vi "Program Setup.vi"(8 "error in (no error)":errorcluster, 10 "shutdown":refnum<user-event>, 11 "Modules":T9) -> (0 "error out":errorcluster)   [LabVIEW 2025]
uses:
  Controls/Sequencer/sequence array.ctl
  Controls/Sequencer/step cluster.ctl
  Controls/Sequencer/action enum.ctl
  Controls/Sequencer/plus button.ctl
  Controls/Sequencer/delete button.ctl
  Controls/Sequencer/save icon.ctl
  Controls/transparent tab control.ctl
  Controls/refresh button 2.ctl
  <vilib>/Handler Framework/CmdQueue/Enqueue Single.vi
  <vilib>/Handler Framework/Handler Framework.lvlib
panel:
  in  "Tab Control":T1
  in  "Refresh":T2
  in  "Program":u16(ring) items=["145", "156", "157", "166", "178"]
  out "View Program Array":T3=[{"Action"=enum."Start", "Angle Min [°]"=0.0, "Angle Max [°]"=0.0, "Torque Min [oz-in]"=0.0, "Torque Max [oz-in]"=0.0}, {"Action"=enum."Return to Home", "Angle Min [°]"=0.0, "Angle Max [°]"=0.0, "Torque Min [oz-in]"=0.0, "Torque Max [oz-in]"=0.0}, {"Action"=enum."End", "Angle Min [°]"=0.0, "Angle Max [°]"=0.0, "Torque Min [oz-in]"=0.0, "Torque Max [oz-in]"=0.0}]
  in  "Array":T3=[{"Action"=enum."Start", "Angle Min [°]"=0.0, "Angle Max [°]"=0.0, "Torque Min [oz-in]"=0.0, "Torque Max [oz-in]"=0.0}, {"Action"=enum."Return to Home", "Angle Min [°]"=0.0, "Angle Max [°]"=0.0, "Torque Min [oz-in]"=0.0, "Torque Max [oz-in]"=0.0}, {"Action"=enum."End", "Angle Min [°]"=0.0, "Angle Max [°]"=0.0, "Torque Min [oz-in]"=0.0, "Torque Max [oz-in]"=0.0}]
  in  "Add Step":T6
  in  "Delete Step":T7
  in  "Save Program":T8
  # "Edit Programs"
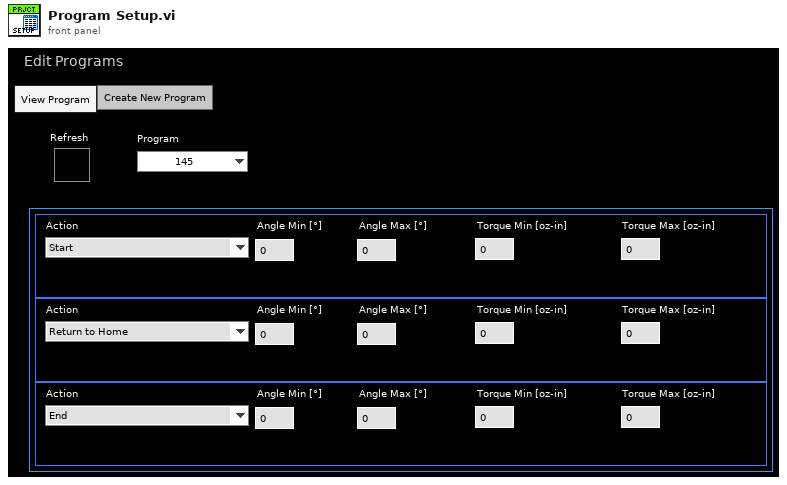
[diagram p1: front panel]
types:
  T1 = typedef "transparent tab control.ctl" = enum32{"View Program", "Create New Program"}
  T2 = typedef "refresh button 2.ctl" = bool
  T3 = typedef "sequence array.ctl" = T4[]
  T4 = typedef "step cluster.ctl" = cluster{"Action":T5, "Angle Min [°]":dbl, "Angle Max [°]":dbl, "Torque Min [oz-in]":dbl, "Torque Max [oz-in]":dbl}
  T5 = typedef "action enum.ctl" = enum16{"Start", "Angle", "Return to Home", "End"}
  T6 = typedef "plus button.ctl" = bool
  T7 = typedef "delete button.ctl" = bool
  T8 = typedef "save icon.ctl" = bool
  T9 = cluster{"Module IDs":i32[], "Module Names":string[]}
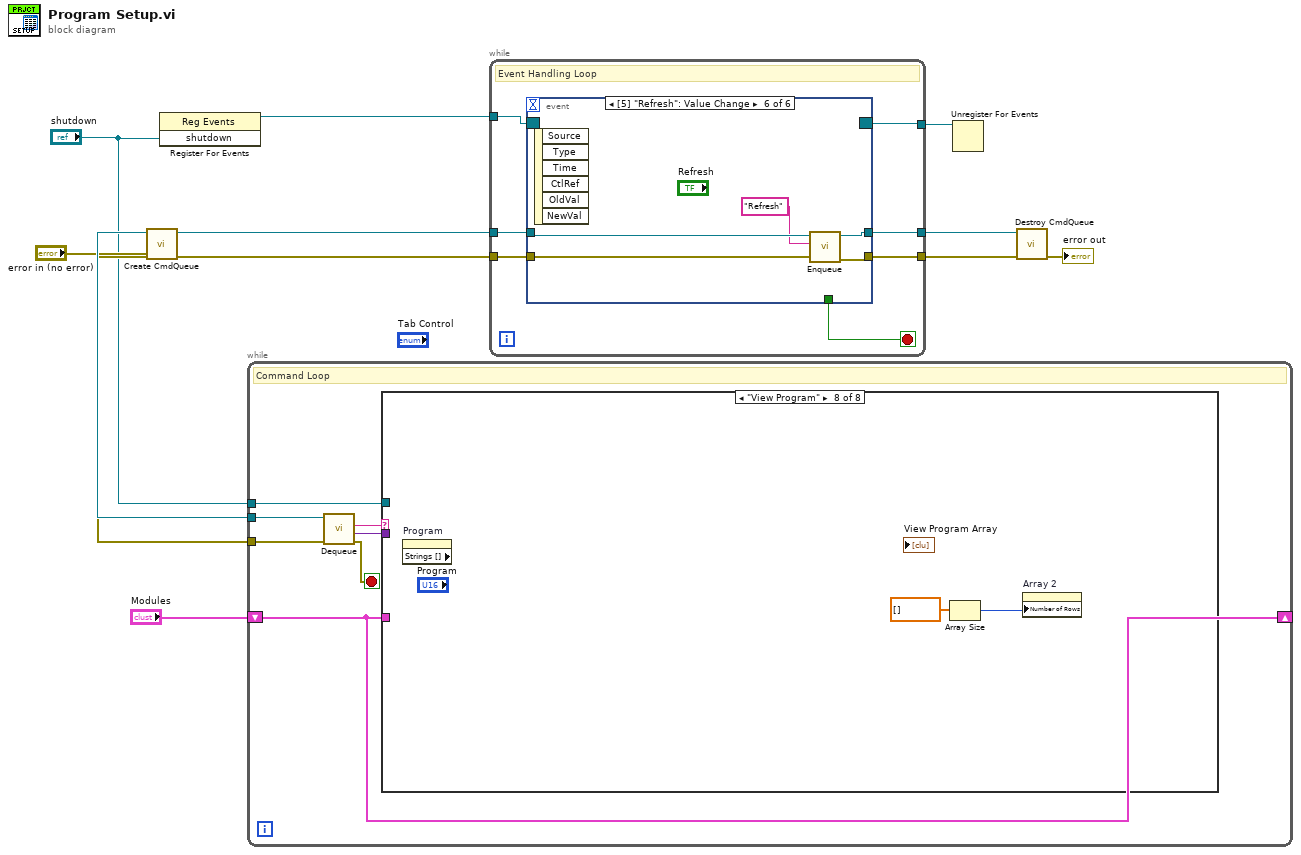
[diagram p0: block diagram]
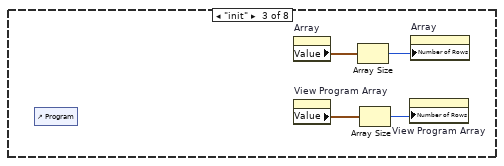
[diagram p4: hidden frame]
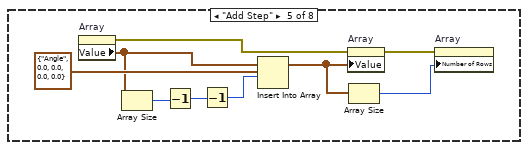
[diagram p6: hidden frame]
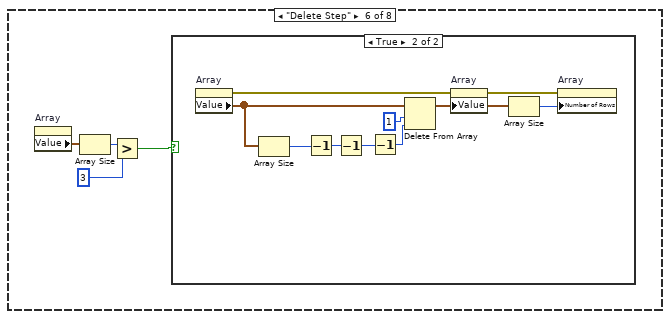
[diagram p7: hidden frame]
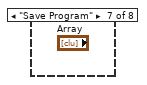
[diagram p9: hidden frame]
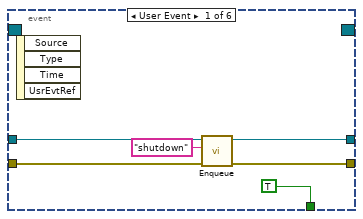
[diagram p10: hidden frame]
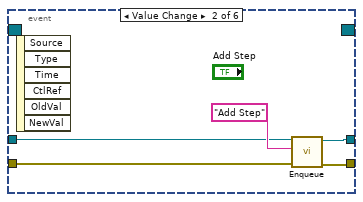
[diagram p11: hidden frame]
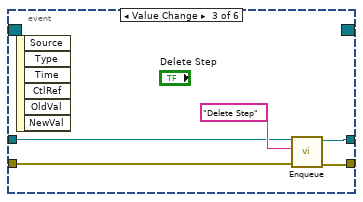
[diagram p12: hidden frame]
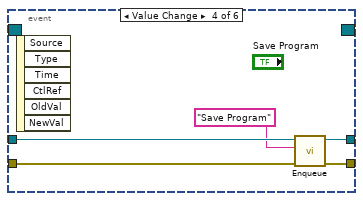
[diagram p13: hidden frame]
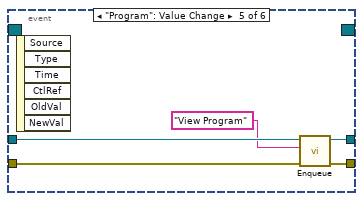
[diagram p14: hidden frame]
diagram:
  n1 = call <vilib>:"Create CmdQueue.vi"("error in (no error)"="error in (no error)") -> ("error out"=w7:errorcluster, "CmdQueue out"=w8:refnum<queue>)  [unwired: 9 in]
  n2 = register-events("shutdown") -> (reference out=w6:refnum<event-registration>)  [unwired: 2 in, 1 out]
  n3 = while {
    tunnel: w8 -> [w17]
    tunnel: w7 -> [w13]
    tunnel: "shutdown" -> [w12]
    shift-right: [w11] -> _
    shift-left: "Modules" -> [w11]
    stop <- w14 stop-if-true
    # "Command Loop"
    n4 = call <vilib>:"Dequeue.vi"("error in (no error)"=w13, "CmdQueue in"=w17) -> ("error out"=w14:errorcluster, "value"=w15:variant, "cmd"=w16:string)  [unwired: 5 in, 2 out]
    n5 = case shown="\"View Program\"" w16 {
      tunnel: w15 -> [_ _ _ _ _ _ _ _]
      tunnel: w12 -> [_ _ _ _ _ _ _ _]
      tunnel: w11 -> [_ _ _ _ _ _ _ _]
      frame "False", Default {
      }
      frame "Refresh" {
      }
      frame "init" {
        n6 = control-ref of="Program"() -> ()  [unwired: 1 out]
        n7 = property on="Array" class="Arr (strict)"() -> ("Value"=w18:T3)  [unwired: 2 in, 2 out]
        n8 = property on="View Program Array" class="Arr (strict)"() -> ("Value"=w20:T3)  [unwired: 2 in, 2 out]
        n9 = Array Size(array=w18) -> (size(s)=w19:i32)
        n10 = Array Size(array=w20) -> (size(s)=w21:i32)
        n11 = property on="View Program Array" class="Arr (strict)"("Number of Rows"=w21) -> ()  [unwired: 2 in, 2 out]
        n12 = property on="Array" class="Arr (strict)"("Number of Rows"=w19) -> ()  [unwired: 2 in, 2 out]
      }
      frame "shutdown" {
      }
      frame "Add Step" {
        n13 = property on="Array" class="Arr (strict)"() -> (error out=w30:errorcluster, "Value"=w23:T3)  [unwired: 2 in, 1 out]
        n14 = Array Size(array=w23) -> (size(s)=w22:i32)
        n15 = Decrement(x=w22) -> (x-1=w29:i32)
        n16 = Decrement(x=w29) -> (x-1=w28:i32)
        n17 = Insert Into Array(array=w23, index=w28, new element=T4 {"Action"=enum."Angle", "Angle Min [°]"=0.0, "Angle Max [°]"=0.0, "Torque Min [oz-in]"=0.0, "Torque Max [oz-in]"=0.0} ("new element/subarray")) -> (w26:T3)
        n18 = property on="Array" class="Arr (strict)"(error in=w30, "Value"=w26) -> (error out=w27:errorcluster)  [unwired: 1 in, 1 out]
        n19 = Array Size(array=w26) -> (size(s)=w25:i32)
        n20 = property on="Array" class="Arr (strict)"(error in=w27, "Number of Rows"=w25) -> ()  [unwired: 1 in, 2 out]
      }
      frame "Delete Step" {
        n21 = property on="Array" class="Arr (strict)"() -> ("Value"=w34:T3)  [unwired: 2 in, 2 out]
        n22 = Array Size(array=w34) -> (size(s)=w33:i32)
        n23 = Greater?(x=w33, y=3) -> (0:w31:bool)
        n24 = case shown="True" w31 {
          frame False {
          }
          frame True {
            n25 = property on="Array" class="Arr (strict)"() -> (error out=w43:errorcluster, "Value"=w37:T3)  [unwired: 2 in, 1 out]
            n26 = Array Size(array=w37) -> (size(s)=w35:i32)
            n27 = Decrement(x=w35) -> (x-1=w36:i32)
            n28 = Decrement(x=w36) -> (x-1=w42:i32)
            n29 = Decrement(x=w42) -> (x-1=w41:i32)
            n30 = Delete From Array(array=w37, length=1, index=w41) -> (array with subset deleted=w39:T3)  [unwired: 1 out]
            n31 = property on="Array" class="Arr (strict)"(error in=w43, "Value"=w39) -> (error out=w40:errorcluster)  [unwired: 1 in, 1 out]
            n32 = Array Size(array=w39) -> (size(s)=w38:i32)
            n33 = property on="Array" class="Arr (strict)"(error in=w40, "Number of Rows"=w38) -> ()  [unwired: 1 in, 2 out]
          }
        }
      }
      frame "Save Program" {
      }
      frame "View Program" {
        n34 = property on="Program" class="Ring (strict)" props=["Strings []"]() -> ()  [unwired: 2 in, 3 out]
        n35 = Array Size(array=dbl[] []) -> (size(s)=w46:i32)
        n36 = property on="Array 2" class="Arr (strict)"("Number of Rows"=w46) -> ()  [unwired: 2 in, 2 out]
      }
    }
  }
  n37 = while {
    tunnel: w8 -> [w53]
    tunnel: [w52] -> w10
    tunnel: w7 -> [w51]
    tunnel: [w50] -> w9
    tunnel: w6 -> [w48]
    tunnel: [w47] -> w5
    stop <- w49 stop-if-true
    # "Event Handling Loop"
    n38 = event shown="[5] \"Refresh\": Value Change" {
      selector: w48 -> [_ _ _ _ _ _]
      dyn-events: [_ _ _ _ _ _] -> w47
      timeout: _ -> [_ _ _ _ _ _]
      tunnel: w53 -> [w59 w61 w66 w72 w77 w82]
      tunnel: [w58 w63 w68 w73 w78 w83] -> w52
      tunnel: w51 -> [w57 w60 w65 w71 w76 w81]
      tunnel: [w56 w64 w69 w74 w79 w84] -> w50
      tunnel: [TRUE ("Discard?") _ _ _ _ _] -> w49
      event User Event {
        n39 = event-data() -> ()  [unwired: 1 in, 4 out]
        n40 = call-poly <vilib>:"Enqueue.vi"("error in (no error)"=w57, "Command"="shutdown", "CmdQueue in"=w59) -> ("error out"=w56:errorcluster, "CmdQueue out"=w58:refnum<queue>)  [unwired: 7 in]
      }
      event Value Change {
        n41 = event-data() -> ()  [unwired: 1 in, 6 out]
        n42 = call-poly <vilib>:"Enqueue.vi"("error in (no error)"=w60, "Command"="Add Step", "CmdQueue in"=w61) -> ("error out"=w64:errorcluster, "CmdQueue out"=w63:refnum<queue>)  [unwired: 7 in]
      }
      event Value Change {
        n43 = event-data() -> ()  [unwired: 1 in, 6 out]
        n44 = call-poly <vilib>:"Enqueue.vi"("error in (no error)"=w65, "Command"="Delete Step", "CmdQueue in"=w66) -> ("error out"=w69:errorcluster, "CmdQueue out"=w68:refnum<queue>)  [unwired: 7 in]
      }
      event Value Change {
        n45 = event-data() -> ()  [unwired: 1 in, 6 out]
        n46 = call-poly <vilib>:"Enqueue.vi"("error in (no error)"=w71, "Command"="Save Program", "CmdQueue in"=w72) -> ("error out"=w74:errorcluster, "CmdQueue out"=w73:refnum<queue>)  [unwired: 7 in]
      }
      event "Program": Value Change {
        n47 = event-data() -> ()  [unwired: 1 in, 6 out]
        n48 = call-poly <vilib>:"Enqueue.vi"("error in (no error)"=w76, "Command"="View Program", "CmdQueue in"=w77) -> ("error out"=w79:errorcluster, "CmdQueue out"=w78:refnum<queue>)  [unwired: 7 in]
      }
      event Value Change {
        n49 = event-data() -> ()  [unwired: 1 in, 6 out]
        n50 = call-poly <vilib>:"Enqueue.vi"("error in (no error)"=w81, "Command"="Refresh", "CmdQueue in"=w82) -> ("error out"=w84:errorcluster, "CmdQueue out"=w83:refnum<queue>)  [unwired: 7 in]
      }
    }
  }
  n51 = Unregister For Events(event registration refnum=w5) -> ()  [unwired: 1 in, 1 out]
  n52 = call <vilib>:"Destroy CmdQueue.vi"("error in (no error)"=w9, "CmdQueue in"=w10) -> ("error out"=→"error out":errorcluster)  [unwired: 9 in]
